vi "LogToXMLFile.vi"(8 "Error In":errorcluster, 11 "Jedi In":refnum<class "Jedi.lvclass">) -> (0 "Error Out":errorcluster, 3 "Jedi Out":refnum<class "Jedi.lvclass">)   [LabVIEW 2021, in "Jedi.lvclass"]
doc: "Save specific class data to file as XML."
uses:
  Jedi.lvclass
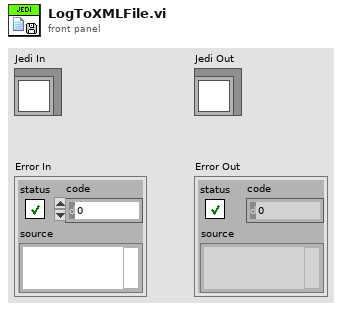
[diagram p1: front panel]
types:
  T1 = enum16{"open", "replace", "create", "open or create", "replace or create", "replace or create with confirmation"}
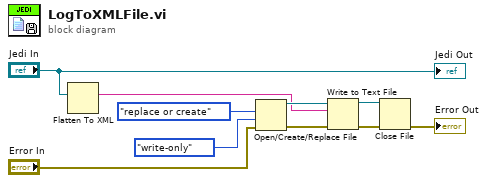
[diagram p0: block diagram]
diagram:
  n1 = Flatten To XML(6:"Jedi In") -> (2:w4:string)
  n2 = Open/Create/Replace File(error in="Error In", operation (0:open)=T1."replace or create", access (0:read/write)=enum16{"read/write", "read-only", "write-only"}."write-only") -> (refnum out=w5:refnum<file>, error out=w6:errorcluster)  [unwired: 3 in, 1 out]
  n3 = Write to Text File(file (use dialog)=w5, text=w4, error in=w6) -> (refnum out=w3:refnum<file>, error out=w2:errorcluster)  [unwired: 1 in, 1 out]
  n4 = Close File(refnum=w3, error in=w2) -> (error out=→"Error Out":errorcluster)  [unwired: 1 out]
  "Jedi Out" <- "Jedi In"
